vi "Show Error Msg.vi"(8 "error in":errorcluster, 10 "Fit to Actor Window":bool, 11 "ViewableActor in":refnum<class "ViewableActor.lvclass">) -> (0 "error out":errorcluster, 3 "ViewableActor out":refnum<class "ViewableActor.lvclass">)   [LabVIEW 2020, in "ViewableActor.lvlib" / "ViewableActor.lvclass"]
uses:
  ViewableActor.lvclass
  C:/Program Files (x86)/National Instruments/LabVIEW 2020/vi.lib/ActorFramework/Actor/Actor.lvclass
  ViewableActor.lvclass/ViewableActor.ctl
  Error Display Actor/Error Display Actor.lvclass
  Error Display Actor/Error Display Actor.lvclass/Error Display Actor.ctl
  ViewableActor Messages/Set IsFrontMost Msg/Set IsFrontMost Msg.lvclass/Set IsFrontMost Msg.ctl
  <vilib>/ActorFramework/Message Enqueuer/Message Enqueuer.lvclass/Message Enqueuer.ctl
  ViewableActor Messages/Shift Window Msg/Shift Window Msg.lvclass/Shift Window Msg.ctl
  Error Display Actor/Write Source Actor.vi
  Error Display Actor/Write error for msg.vi
  Read Actor Name.vi
  <vilib>/ActorFramework/Message Enqueuer/Enqueue.vi
  ViewableActor Messages/Set IsFrontMost Msg/Set IsFrontMost Msg.lvclass
  C:/Program Files (x86)/National Instruments/LabVIEW 2020/vi.lib/ActorFramework/Message/Message.lvclass
  ViewableActor Messages/Open Front Panel Msg/Open Front Panel Msg.lvclass
  ViewableActor Messages/Shift Window Msg/Shift Window Msg.lvclass
  <vilib>/ActorFramework/Message Priority Queue/Priority Enqueue.vi
  <vilib>/ActorFramework/Actor/Actor.lvclass
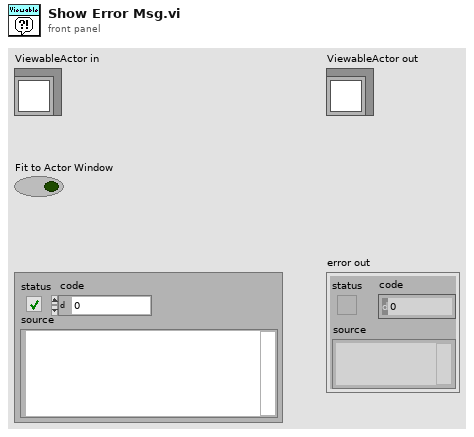
[diagram p1: front panel]
types:
  T1 = typedef "LVPositionTypeDef.ctl" = cluster{"Left":i32, "Top":i32}
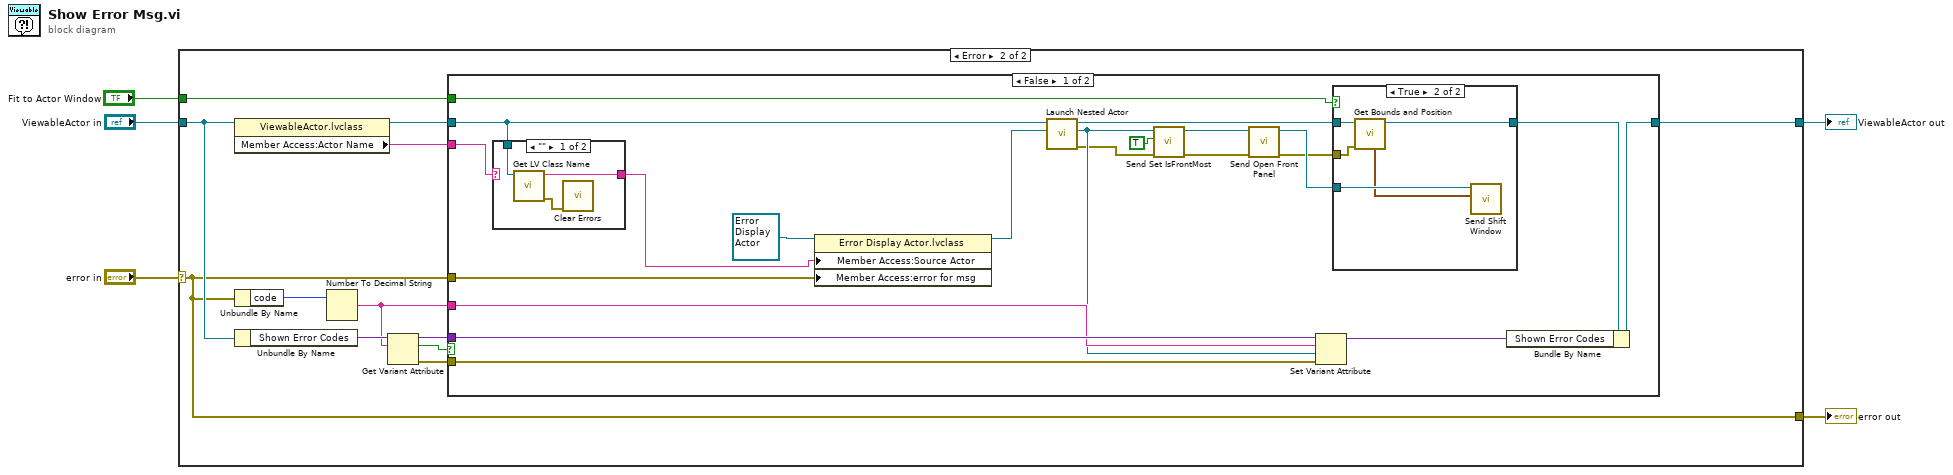
[diagram p0: block diagram]
diagram:
  n1 = case shown="Error" "error in" {
    selector: "error in" -> [w6 w11]
    tunnel: [w6 w11] -> w4
    tunnel: [w7 w17] -> w2
    tunnel: "ViewableActor in" -> [w7 w16]
    tunnel: "Fit to Actor Window" -> [_ w8]
    frame No Error {
      # "Wire the error cluster across even in the \"No Error\"\ncase so that warnings get propagated."
    }
    frame Error {
      n2 = property class="ViewableActor.lvclass"(reference=w16) -> (reference out=w18:refnum<class "ViewableActor.lvclass">, "Member Access:Actor Name"=w19:string)  [unwired: 1 in, 1 out]
      n3 = Unbundle By Name(w11) -> ("code"=w14:i32)
      n4 = Unbundle By Name(w16) -> ("Shown Error Codes"=w15:variant)
      n5 = Number To Decimal String(number=w14) -> (decimal integer string=w9:string)  [unwired: 1 in]
      n6 = Get Variant Attribute(Variant=w15, name=w9) -> (duplicate Variant=w12:variant, found=w13:bool, error out=w10:errorcluster)  [unwired: 2 in, 1 out]
      n7 = case shown="False" w13 {
        tunnel: w19 -> [w40 _]
        tunnel: w18 -> [w32 w51]
        tunnel: [w38 w51] -> w17
        tunnel: w12 -> [w37 _]
        tunnel: w11 -> [w35 _]
        tunnel: w10 -> [w34 _]
        tunnel: w9 -> [w30 _]
        tunnel: w8 -> [w28 _]
        frame False {
          n8 = case shown="\"\"" w40 {
            selector: w40 -> [_ w50]
            tunnel: [w48 w50] -> w20
            tunnel: w32 -> [w49 _]
            frame "" {
              n9 = call <vilib>:"Get LV Class Name.vi"("object"=w49) -> ("error out"=w47:errorcluster, "class name"=w48:string)  [unwired: 9 in]
              n10 = call <vilib>:"Clear Errors.vi"("error in (no error)"=w47) -> ()  [unwired: 5 in, 2 out]
            }
            frame Default {
            }
          }
          n11 = property class="Error Display Actor.lvclass"(reference=refnum<class "Error Display Actor.lvclass"> refnum ("ViewableActor.lvlib:Error Display Actor.lvclass"), "Member Access:Source Actor"=w20, "Member Access:error for msg"=w35) -> (reference out=w31:refnum<class "Error Display Actor.lvclass">)  [unwired: 1 in, 1 out]
          n12 = call <vilib>:"Launch Nested Actor.vi"("Nested Actor"=w31, "Caller Actor in"=w32) -> ("error out"=w22:errorcluster, "Nested Actor's Enqueuer"=w27:refnum<class "Message Enqueuer.lvclass">, "Caller Actor out"=w33:refnum<class "ViewableActor.lvclass">)  [unwired: 7 in]
          n13 = call "Send Set IsFrontMost.vi"("error in (no error)"=w22, "IsFrontMost"=TRUE, "Message Enqueuer"=w27) -> ("error out"=w21:errorcluster, "Message Enqueuer out"=w24:refnum<class "Message Enqueuer.lvclass">)  [unwired: 7 in]
          n14 = call "Send Open Front Panel.vi"("error in (no error)"=w21, "Message Enqueuer"=w24) -> ("error out"=w25:errorcluster, "Message Enqueuer out"=w26:refnum<class "Message Enqueuer.lvclass">)  [unwired: 8 in]
          n15 = Set Variant Attribute(Variant=w37, name=w30, value=w27, error in=w34) -> (Variant out=w29:variant)  [unwired: 2 out]
          n16 = case shown="True" w28 {
            tunnel: [w41 w46] -> w39
            tunnel: w33 -> [w41 w45]
            tunnel: w25 -> [_ w44]
            tunnel: w26 -> [_ w43]
            frame False {
            }
            frame True {
              n17 = call-dynamic "Get Bounds and Position.vi"("error in (no error)"=w44, "ViewableActor in"=w45) -> ("ViewableActor out"=w46:refnum<class "ViewableActor.lvclass">, "Panel Position"=w42:T1)  [unwired: 5 in, 3 out]
              n18 = call "Send Shift Window.vi"("top left point"=w42, "Message Enqueuer"=w43) -> ()  [unwired: 8 in, 2 out]
            }
          }
          n19 = Bundle By Name(cluster=w39, "Shown Error Codes"=w29) -> (w38:refnum<class "ViewableActor.lvclass">)
        }
        frame True {
          # "#30.04.2025 Der Fehler wird bereits angezeigt, ignoriere"
        }
      }
    }
  }
  "error out" <- w4
  "ViewableActor out" <- w2
